vi "Picolog Read Channel.vi"(8 "Error In":errorcluster, 10 "Units":T1, 11 "Instrument Handle In":i16) -> (0 "Error Out":errorcluster, 2 "Temperature buffer":dbl[](array[numeric]), 3 "Instrument Handle Out":i16)   [LabVIEW 2016]
uses:
  Controls/Temperature Units.ctl
  usbtc08.dll
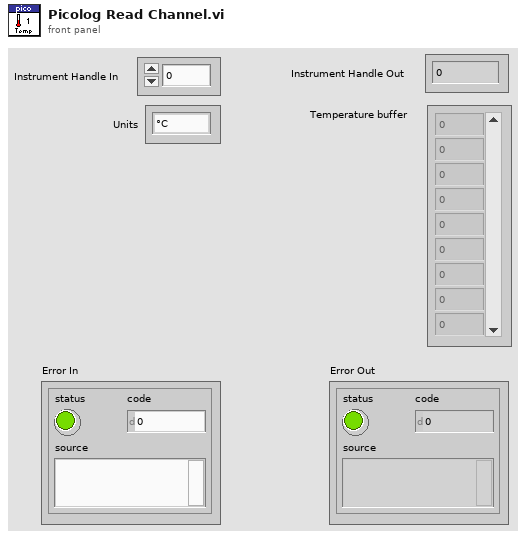
[diagram p1: front panel]
types:
  T1 = typedef "Temperature Units.ctl" = enum16{"°C", "°F", "K", "°R"}
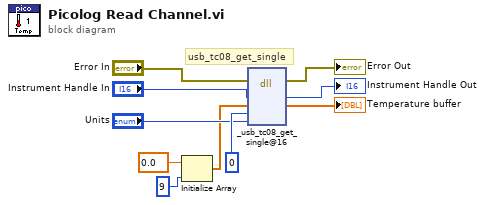
[diagram p0: block diagram]
diagram:
  # "usb_tc08_get_single"
  n1 = Initialize Array(sgl 0.0, i16 9) -> (w4:sgl[])
  n2 = dll-call lib="usbtc08.dll" fn="_usb_tc08_get_single@16"(error in="Error In", "handle"="Instrument Handle In", "temp_buffer"=w4, "overflow"=i16 0, "units"="Units") -> (error out=→"Error Out":errorcluster, "handle"=→"Instrument Handle Out":i16, "temp_buffer"=→"Temperature buffer":sgl[])  [unwired: 5 in, 1 out]
